vi "TF_Encoder2PositionEndEffector.vi"(0 "Divide":dbl, 2 "Counter Value":i32, 4 "Offset":dbl) -> (5 "Position [deg]":dbl format="%#_13g")   [LabVIEW 2015]
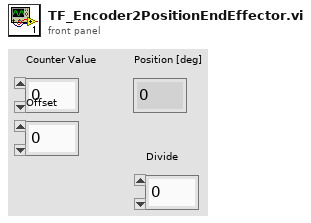
[diagram p1: front panel]
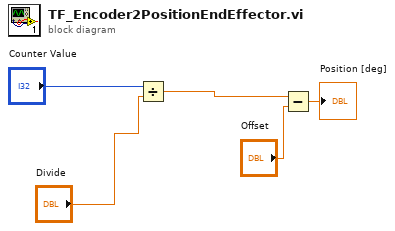
[diagram p0: block diagram]
diagram:
  n1 = Divide(x="Counter Value", y="Divide") -> (x/y=w1:dbl)
  n2 = Subtract(x=w1, y="Offset") -> (x-y=→"Position [deg]":dbl)
